vi "AbberationList_ae.vi"(1 "Enum":enum16{"WRITE", "READ"}(ring), 7 "Abberation Cluster In":T1) -> (8 "Abberation Cluster Out":T1)   [LabVIEW 2014]
uses:
  AbberationControl.ctl
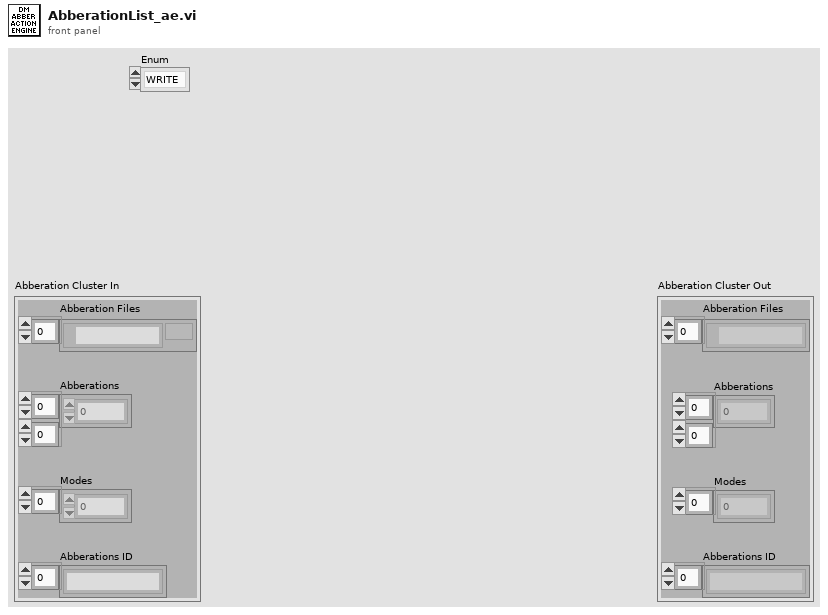
[diagram p1: front panel]
types:
  T1 = typedef "AbberationControl.ctl" = cluster{"Abberations":dbl[][], "Modes":i32[], "Abberations ID":string[], "Abberation Files":path[]}
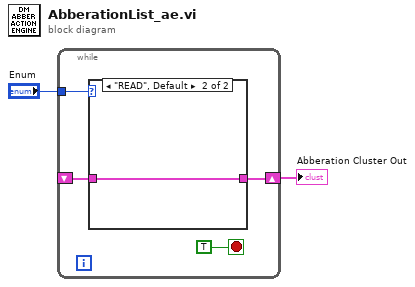
[diagram p0: block diagram]
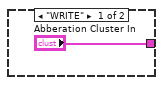
[diagram p2: hidden frame]
diagram:
  n1 = while {
    tunnel: "Enum" -> [w5]
    shift-right: [w4] -> w1
    shift-left: _ -> [w3]
    stop <- TRUE stop-if-true
    n2 = case shown="\"READ\", Default" w5 {
      tunnel: ["Abberation Cluster In" w8] -> w4
      tunnel: w3 -> [_ w8]
      frame "WRITE" {
      }
      frame "READ", Default {
      }
    }
  }
  "Abberation Cluster Out" <- w1
